vi "climber.vi"(9 "Climber Down":bool, 10 "Climber Up":bool) -> ()   [LabVIEW 2020]
uses:
  <vilib>/Rock Robotics/WPI/ThirdParty/Phoenix-LabVIEW/Motor Controller/Controls/CTRE_Phoenix_MotorControl_ControlMode.ctl
  TitanLib/Lib/Piston Hold.vi
  <vilib>/Rock Robotics/WPI/Solenoid/WPI_SolenoidSetEnum.vi
  TitanLib/Lib/TitanLib.lvlib
panel:
  in  "Zero Encoders":bool
  in  "Climber Manual Power":dbl=0.25
  in  "Climber Manual Override?":bool=TRUE
  in  "Climber Up Pos":dbl=-9.82
  in  "Climber Down Pos":dbl=-0.5
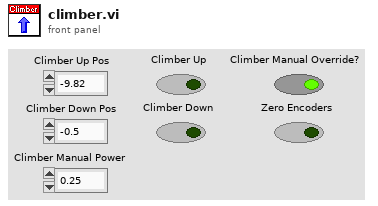
[diagram p1: front panel]
types:
  T1 = typedef "WPI_MotorControlDeviceRef.ctl" = cluster{"DeviceStatus":errorcluster, "Type":T2, "PWM":cluster{"PWM Channel":T3, "DeadBand":T4}, "CAN":cluster{"Device Number":u8, "SetOutput VI Ref":variant, "GetOutput VI Ref":variant, "Enable VI Ref":variant, "Disable VI Ref":variant, "Data":variant}, "Invert":bool, "DIO PWM":cluster{"PWM \"Enable\" Channel":T3, "DIOChannel":T5, "PWM Rate":dbl}}
  T2 = typedef "WPI_MotorControlType.ctl" = enum16{"PWM", "CAN", "DIO PWM"}
  T3 = typedef "FPGA_DIOPWMChannel.ctl" = enum8{"PWM 0", "PWM 1", "PWM 2", "PWM 3", "PWM 4", "PWM 5", "PWM 6", "PWM 7", "PWM 8", "PWM 9", "PWM MXP 0", "PWM MXP 1", "PWM MXP 2", "PWM MXP 3", "PWM MXP 4", "PWM MXP 5", "PWM MXP 6", "PWM MXP 7", "PWM MXP 8", "PWM MXP 9", "Invalid"}
  T4 = typedef "WPI_PWMDeadband.ctl" = cluster{"Name":string, "maxPositivePwm":i32, "minPositivePwm":i32, "centerPwm":i32, "maxNegativePwm":i32, "minNegativePwm":i32, "angularRange":u16}
  T5 = typedef "FPGA_DIOChannel.ctl" = enum8{"DIO 0", "DIO 1", "DIO 2", "DIO 3", "DIO 4", "DIO 5", "DIO 6", "DIO 7", "DIO 8", "DIO 9", "DIO MXP 0", "DIO MXP 1", "DIO MXP 2", "DIO MXP 3", "DIO MXP 4", "DIO MXP 5", "DIO MXP 6", "DIO MXP 7", "DIO MXP 8", "DIO MXP 9", "DIO MXP 10", "DIO MXP 11", "DIO MXP 12", "DIO MXP 13", "DIO MXP 14", "DIO MXP 15", "SPI Port CS1", "SPI Port CS2", "SPI Port CS3", "SPI Port MISO", "SPI Port MOSI", "Invalid"}
  T6 = typedef "CTRE_Phoenix_MotorControl_ControlMode.ctl" = u16
  T7 = typedef "WPI_SolenoidValue.ctl" = enum16{"Off", "On", "Forward", "Reverse"}
  T8 = typedef "WPI_SolenoidDevRef.ctl" = cluster{"DevStatus":errorcluster, "Pneumatics Control Module":u8, "Forward Solenoid Channel":T9, "Reverse Solenoid Channel":T9}
  T9 = typedef "WPI_SolenoidChannel.ctl" = enum8{"Solenoid 0", "Solenoid 1", "Solenoid 2", "Solenoid 3", "Solenoid 4", "Solenoid 5", "Solenoid 6", "Solenoid 7", "Solenoid 8", "Solenoid 9", "Solenoid 10", "Solenoid 11", "Solenoid 12", "Solenoid 13", "Solenoid 14", "Solenoid 15", "Invalid"}
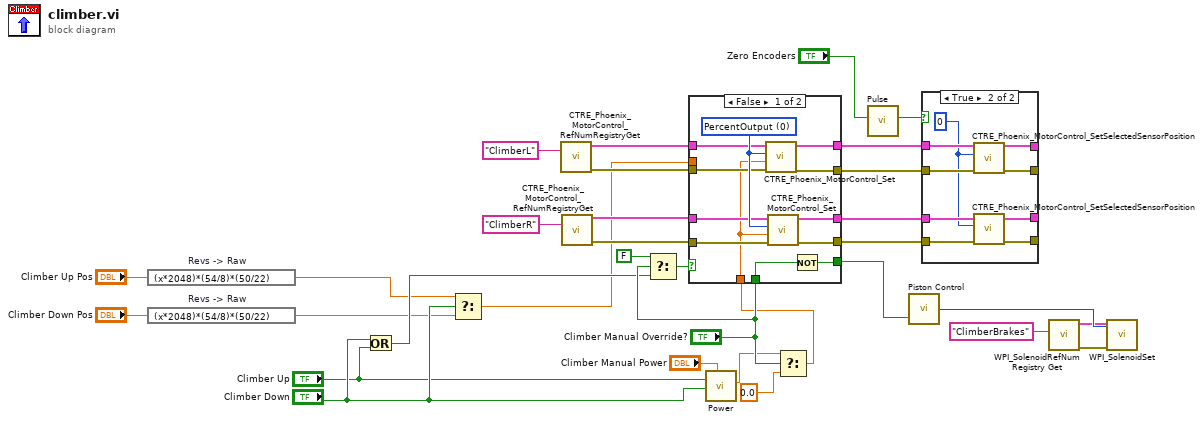
[diagram p0: block diagram]
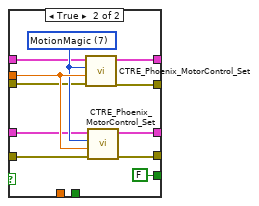
[diagram p3: hidden frame]
diagram:
  n1 = expression code="(x*2048)*(54/8)*(50/22)" "Revs -> Raw"("Climber Up Pos") -> (w2:dbl)
  n2 = expression code="(x*2048)*(54/8)*(50/22)" "Revs -> Raw"("Climber Down Pos") -> (w1:dbl)
  n3 = Or(x="Climber Down", y="Climber Up") -> (x .or. y?=w17:bool)
  n4 = Select(t=w2, s="Climber Down", f=w1) -> (s? t:f=w12:dbl)
  n5 = call <vilib>:"CTRE_Phoenix_MotorControl_RefNumRegistryGet.vi"("refnum name"="ClimberL") -> ("error out"=w26:errorcluster, "PhoenixMotorControlDevRef"=w25:T1)  [unwired: 9 in]
  n6 = call <vilib>:"CTRE_Phoenix_MotorControl_RefNumRegistryGet.vi"("refnum name"="ClimberR") -> ("error out"=w28:errorcluster, "PhoenixMotorControlDevRef"=w27:T1)  [unwired: 9 in]
  n7 = Select(t=FALSE, s="Climber Manual Override?", f=w17) -> (s? t:f=w16:bool)
  n8 = call "Power.vi"("Positive Power"="Climber Manual Power", "Negative"="Climber Up", "Positive"="Climber Down") -> ("Output"=w13:dbl)  [unwired: 8 in]
  n9 = Select(t=w13, s="Climber Manual Override?", f=0.0 ("Output")) -> (s? t:f=w15:dbl)
  n10 = case shown="False" w16 {
    tunnel: w12 -> [_ w55]
    tunnel: w25 -> [w43 w53]
    tunnel: w27 -> [w41 w52]
    tunnel: w28 -> [w40 w51]
    tunnel: w26 -> [w42 w50]
    tunnel: w15 -> [w39 _]
    tunnel: [w38 w49] -> w6
    tunnel: [w37 w48] -> w7
    tunnel: [w36 w47] -> w8
    tunnel: [w35 w46] -> w9
    tunnel: [w34 FALSE ("t")] -> w23
    tunnel: "Climber Manual Override?" -> [w33 _]
    frame False {
      w44 = T6 0 items=["PercentOutput"=0, "Position"=1, "Velocity"=2, "Current"=3, "Follower"=5, "MotionProfile"=6, "MotionMagic"=7, "MotionProfileArc"=10, "Disabled"=15] ("Control Mode")
      n11 = call <vilib>:"CTRE_Phoenix_MotorControl_Set.vi"("error in (no error)"=w42, "Output"=w39, "Control Mode"=w44, "PhoenixMotorControlDevRef"=w43) -> ("error out"=w37:errorcluster, "PhoenixMotorControlDevRef"=w38:T1)  [unwired: 6 in]
      n12 = call <vilib>:"CTRE_Phoenix_MotorControl_Set.vi"("error in (no error)"=w40, "Output"=w39, "Control Mode"=w44, "PhoenixMotorControlDevRef"=w41) -> ("error out"=w35:errorcluster, "PhoenixMotorControlDevRef"=w36:T1)  [unwired: 6 in]
      n13 = Not(x=w33) -> (.not. x?=w34:bool)
    }
    frame True {
      w54 = T6 7 items=["PercentOutput"=0, "Position"=1, "Velocity"=2, "Current"=3, "Follower"=5, "MotionProfile"=6, "MotionMagic"=7, "MotionProfileArc"=10, "Disabled"=15] ("Control Mode")
      n14 = call <vilib>:"CTRE_Phoenix_MotorControl_Set.vi"("error in (no error)"=w50, "Output"=w55, "Control Mode"=w54, "PhoenixMotorControlDevRef"=w53) -> ("error out"=w48:errorcluster, "PhoenixMotorControlDevRef"=w49:T1)  [unwired: 6 in]
      n15 = call <vilib>:"CTRE_Phoenix_MotorControl_Set.vi"("error in (no error)"=w51, "Output"=w55, "Control Mode"=w54, "PhoenixMotorControlDevRef"=w52) -> ("error out"=w46:errorcluster, "PhoenixMotorControlDevRef"=w47:T1)  [unwired: 6 in]
    }
  }
  n16 = call "Pulse.vi"("Input"="Zero Encoders") -> ("Output"=w10:bool)  [unwired: 10 in]
  n17 = call-poly "Piston Control.vi"("Input"=w23) -> ("Output"=w22:T7)  [unwired: 1 in]
  n18 = case shown="True" w10 {
    tunnel: w6 -> [w59 w68]
    tunnel: w7 -> [w58 w67]
    tunnel: w8 -> [w57 w66]
    tunnel: w9 -> [w56 w65]
    tunnel: [w59 w63] -> _
    tunnel: [w58 w62] -> _
    tunnel: [w57 w61] -> _
    tunnel: [w56 w60] -> _
    frame False {
    }
    frame True {
      w64 = 0 ("New Sensor Position")
      n19 = call <vilib>:"CTRE_Phoenix_MotorControl_SetSelectedSensorPosition.vi"("error in (no error)"=w67, "New Sensor Position"=w64, "PhoenixMotorControlDevRef"=w68) -> ("error out"=w62:errorcluster, "PhoenixMotorControlDevRef"=w63:T1)  [unwired: 7 in]
      n20 = call <vilib>:"CTRE_Phoenix_MotorControl_SetSelectedSensorPosition.vi"("error in (no error)"=w65, "New Sensor Position"=w64, "PhoenixMotorControlDevRef"=w66) -> ("error out"=w60:errorcluster, "PhoenixMotorControlDevRef"=w61:T1)  [unwired: 7 in]
    }
  }
  n21 = call <vilib>:"WPI_SolenoidRefNum Registry Get.vi"("refnum name"="ClimberBrakes") -> ("error out"=w20:errorcluster, "SolenoidDevRef"=w19:T8)  [unwired: 9 in]
  n22 = call-poly <vilib>:"WPI_SolenoidSet.vi"("error in (no error)"=w20, "Value"=w22, "SolenoidDevRef"=w19) -> ()  [unwired: 7 in, 2 out]
